vi "Filter Resource VIs.vi"(8 "Error In":errorcluster, 11 "VIs In":T1[](array[typedef])) -> (0 "Error Out":errorcluster, 3 "VIs Out":T1[](array[typedef]))   [LabVIEW 2018, in "Bookmark Manager.lvlib"]
uses:
  Bookmark Manager.lvlib
  Controls/BMark_VI_Identifier.ctl
  <vilib>/addons/analyzer/_analyzerctrls.llb/VIAnCtl Analysis App Info.ctl
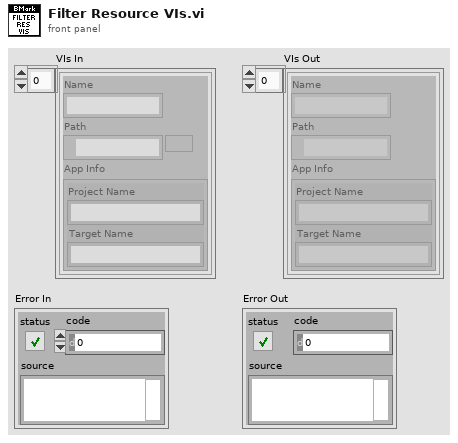
[diagram p1: front panel]
types:
  T1 = typedef "Bookmark Manager.lvlib/BMark_VI_Identifier.ctl" = cluster{"Name":string, "Path":path, "App Info":T2}
  T2 = typedef "VIAnCtl Analysis App Info.ctl" = cluster{"Project Name":string, "Target Name":string}
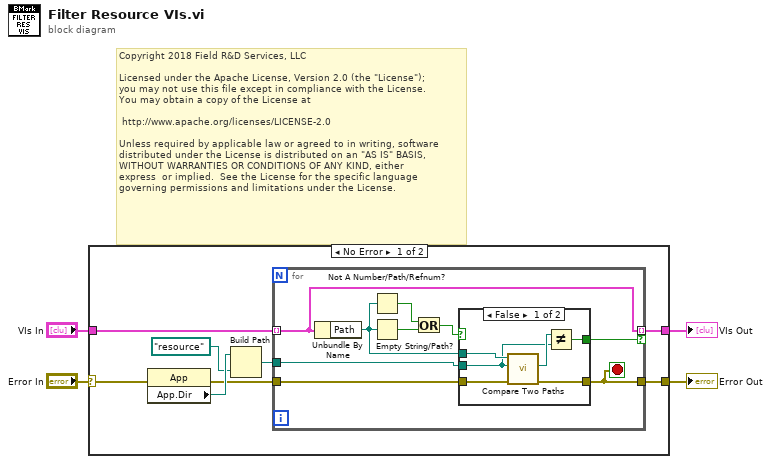
[diagram p0: block diagram]
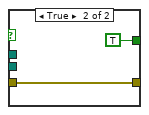
[diagram p2: hidden frame]
diagram:
  # "Copyright 2018 Field R&D Services, LLC\n\nLicensed under the Apache License, Version 2.0 (the \"License\");\nyou may not use this file except in compliance with the License.\nYou may obtain a copy of the License at\n\n\thttp://www.apache.org/licenses/LICENSE-2.0\n\nUnless required by applicable law or agreed to in writing, software\ndistributed under the License is distributed on an \"AS IS\" BASIS,\nWITHOUT WARRANTIES OR CONDITIONS OF ANY KIND, either \nexpress  or implied.  See the License for the specific language \ngoverning permissions and limitations under the License."
  n1 = case shown="No Error" "Error In" {
    selector: "Error In" -> [w6 w31]
    tunnel: [w12 w31] -> w4
    tunnel: "VIs In" -> [w11 w30]
    tunnel: [w10 w30] -> w1
    frame No Error {
      n2 = property class="App"(error in=w6) -> (error out=w5:errorcluster, "App.Dir"=w9:path)  [unwired: 1 in, 1 out]
      n3 = Build Path(base path=w9, name or relative path=path "resource") -> (appended path=w7:path)
      n4 = for {
        tunnel: w11 -> [w20] mode=indexing
        tunnel: w5 -> [w21]
        tunnel: [w18] -> w12
        tunnel: [w20] -> w10 mode=indexing if=w19
        tunnel: w7 -> [w17]
        stop <- w18 stop-if-true
        n5 = Unbundle By Name(w20) -> ("Path"=w14:path)
        n6 = Not A Number/Path/Refnum?(number/path/refnum=w14) -> (NaN/Path/Refnum?=w16:bool)
        n7 = Empty String/Path?(string/path=w14) -> (empty?=w15:bool)
        n8 = Or(x=w16, y=w15) -> (x .or. y?=w13:bool)
        n9 = case shown="False" w13 {
          tunnel: w14 -> [w27 _]
          tunnel: w21 -> [w26 w29]
          tunnel: [w25 w29] -> w18
          tunnel: [w23 TRUE] -> w19
          tunnel: w17 -> [w22 _]
          frame False {
            n10 = call <vilib>:"Compare Two Paths.vi"("error in (no error)"=w26, "Path 2"=w22, "Path 1"=w27) -> ("error out"=w25:errorcluster, "Common Path"=w24:path)  [unwired: 5 in, 2 out]
            n11 = Not Equal?(x=w24, y=w22) -> (x != y?=w23:bool)
          }
          frame True {
          }
        }
      }
    }
    frame Error {
    }
  }
  "Error Out" <- w4
  "VIs Out" <- w1
